vi "Setup subWorker - LoginView.vi"(8 "error in":errorcluster, 11 "Manager Panel in":refnum<class "Manager Panel.lvclass">) -> (0 "error out":errorcluster, 3 "Manager Panel out":refnum<class "Manager Panel.lvclass">)   [LabVIEW 2020, in "Manager Panel.lvclass"]
doc: "This VI sets up the framework parameters of a statically-linked subWorker."
uses:
  Manager Panel.lvclass
  Manager Panel.lvclass/Manager Panel.ctl
  LoginView/LoginView.lvclass
  C:/Program Files (x86)/National Instruments/LabVIEW 2020/vi.lib/addons/_Workers/Library/Classes/Worker/Worker.lvclass
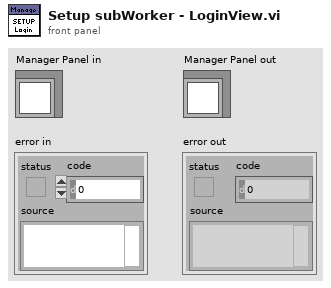
[diagram p1: front panel]
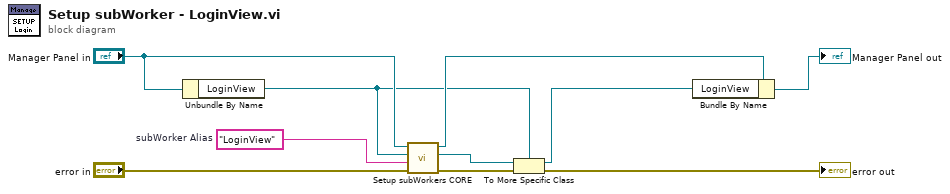
[diagram p0: block diagram]
diagram:
  w6 = "LoginView"  # subWorker Alias
  n1 = Unbundle By Name("Manager Panel in") -> ("LoginView"=w3:refnum<class "LoginView.lvclass">)
  n2 = call-dynamic "Setup subWorkers CORE.vi"("error in"="error in", "subWorker Alias"=w6, "subWorker"=w3, "Worker"="Manager Panel in") -> ("error out"=w5:errorcluster, "subWorker out"=w1:refnum<class "Worker.lvclass">, "Worker out"=w8:refnum<class "Manager Panel.lvclass">)  [unwired: 5 in]
  n3 = To More Specific Class(target class=w3, reference=w1, error in=w5) -> (specific class reference=w2:refnum<class "LoginView.lvclass">, error out=→"error out":errorcluster)
  n4 = Bundle By Name(cluster=w8, "LoginView"=w2) -> (→"Manager Panel out":refnum<class "Manager Panel.lvclass">)
